vi "Full Cholesky Factorization.vi"   [LabVIEW 2017, in "NI_AALBase.lvlib"]
uses:
  <vilib>/Analysis/NI_AALBase.lvlib
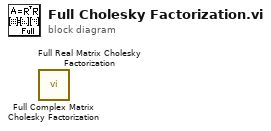
[diagram p0: block diagram]
diagram:
  n1 = call <vilib>:"Full Complex Matrix Cholesky Factorization.vi"() -> ()  [unwired: 1 in, 2 out]
  n2 = call <vilib>:"Full Real Matrix Cholesky Factorization.vi"() -> ()  [unwired: 1 in, 2 out]
